vi "Run.vi"(11 "error in":errorcluster) -> (15 "error out":errorcluster)   [LabVIEW 2016, in "CarWashTest.lvlib"]
uses:
  CarWashTest.lvlib
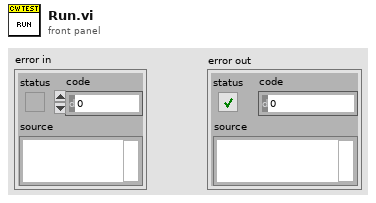
[diagram p1: front panel]
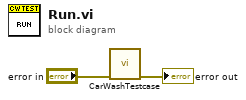
[diagram p0: block diagram]
diagram:
  n1 = call "CarWashTestcase.vi"("error in"="error in") -> ("error out"=→"error out":errorcluster)  [unwired: 14 in]
